vi "NurseStationMain.vi"() -> ()   [LabVIEW 2015]
uses:
  TypeDef/SelectedRoom.ctl
  LVClasses/Flags/ColorFlags.ctl
  TypeDef/RoomSelFromMap.ctl
  TypeDef/Flags_RoomNumber.ctl
  LVClasses/Room/Room.lvclass/Room.ctl
  TypeDef/State Cluster.ctl
  LVClasses/Room/Room.lvclass
  LVRestAPI/TypeDef/FGVAction.ctl
  LVClasses/Room/Read Flags.lvclass.vi
  LVClasses/Room/Read Room Number.vi
  LVClasses/Flags/Flags.lvclass
  LVRestAPI/RestApi.lvlib
panel:
  in  "Tab Control":enum32{"Main View", "Reports", "Debug"}(tab)
  out "Rooms":T1[](array[typedef])
  in  "New Request":bool
  out "Selected Room":T3={"Room Number"=0, "RoomNumFlags"={"Flag State"=[1, 3, 5, 7]}, "BedVacant"=FALSE, "InRoomPersonnel"=[], "RoomRequests"=[]}
  in  "SelRoom101":T4
  in  "SelRoom102":T4
  in  "SelRoom103":T4
  in  "stop":bool
  in  "ClearRequest":bool
  in  "ReqIndex":i32
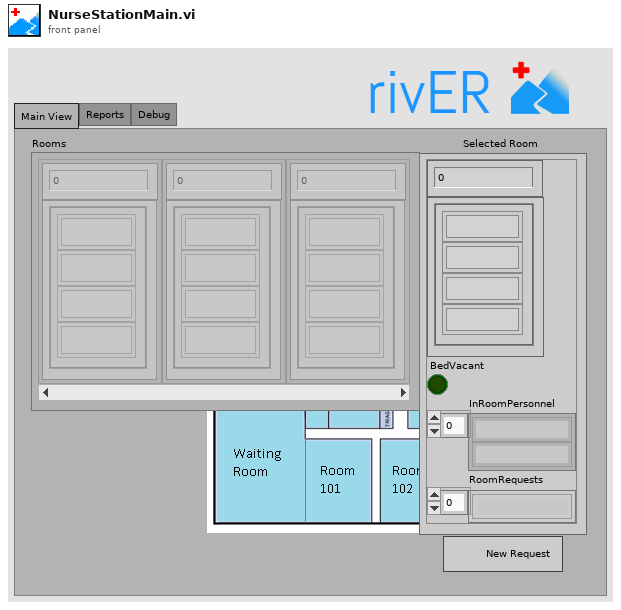
[diagram p1: front panel]
types:
  T1 = typedef "Flags_RoomNumber.ctl" = cluster{"Room Number":i32, "RoomNumFlags":T2}
  T2 = typedef "Flags.lvclass/ColorFlags.ctl" = cluster{"Flag State":u8[]}
  T3 = typedef "SelectedRoom.ctl" = cluster{"Room Number":u8, "RoomNumFlags":T2, "BedVacant":bool, "InRoomPersonnel":string[], "RoomRequests":string[]}
  T4 = typedef "RoomSelFromMap.ctl" = bool
  T5 = typedef "EventsReference.ctl" = cluster{"Init":refnum<user-event>, "Refresh UI":refnum<user-event>}
  T6 = typedef "FGVAction.ctl" = enum16{"Get", "Set"}
  T7 = typedef "State Cluster.ctl" = cluster{"Room Array":refnum<class "Room.lvclass">[], "Selected Room":u32}
  T8 = typedef "LVPoint32TypeDef.ctl" = cluster{"Horizontal":i32, "Vertical":i32}
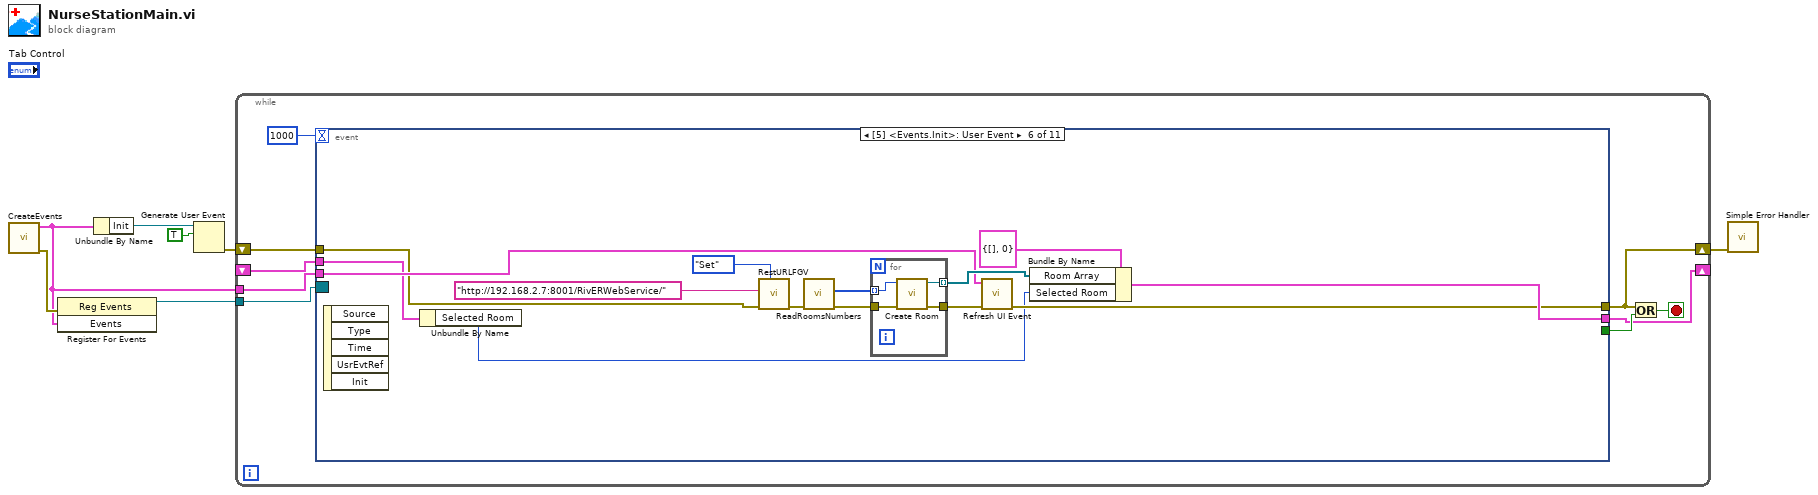
[diagram p0: block diagram]
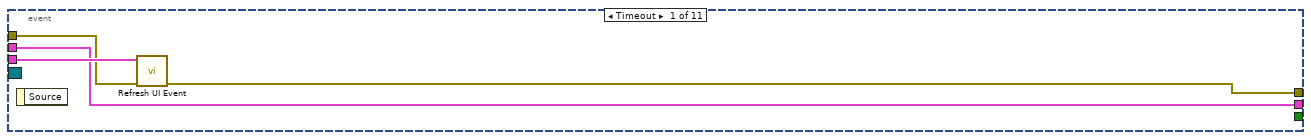
[diagram p2: hidden frame]
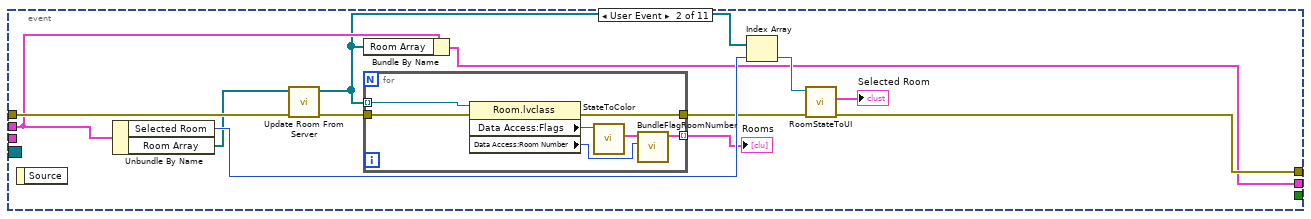
[diagram p3: hidden frame]
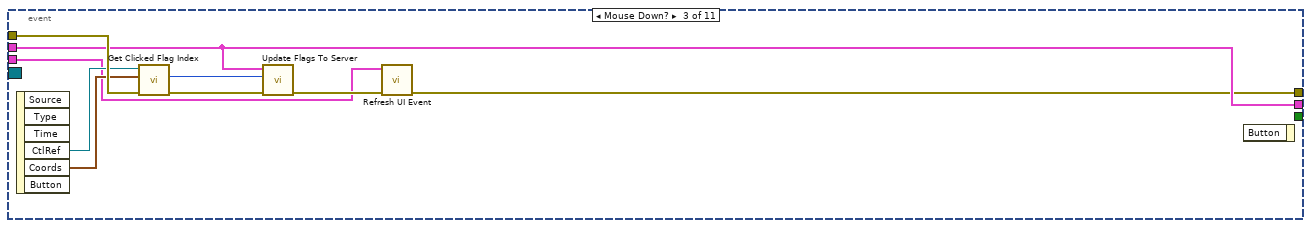
[diagram p4: hidden frame]
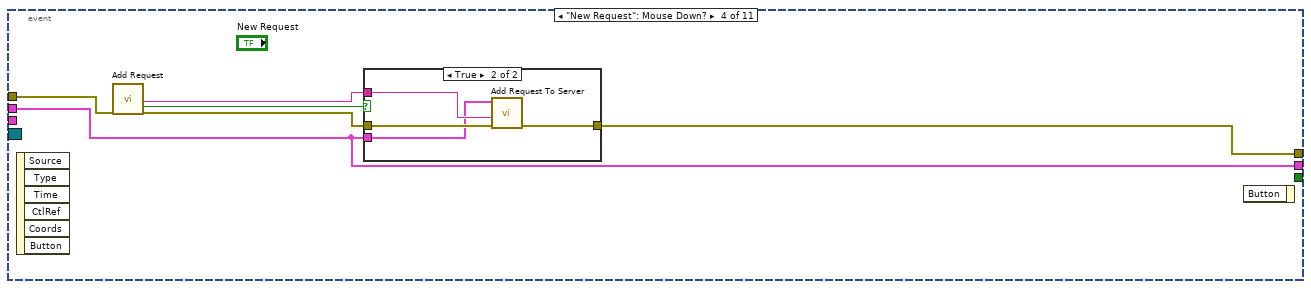
[diagram p5: hidden frame]
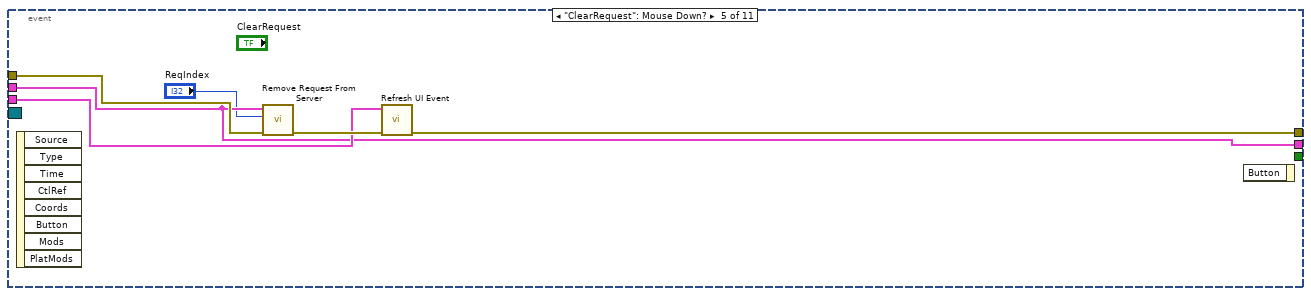
[diagram p7: hidden frame]
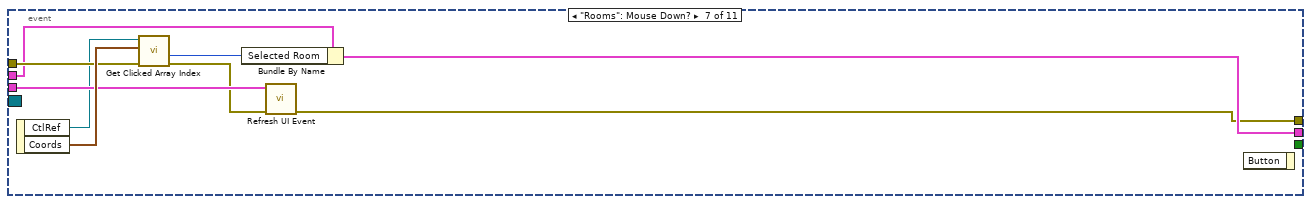
[diagram p8: hidden frame]
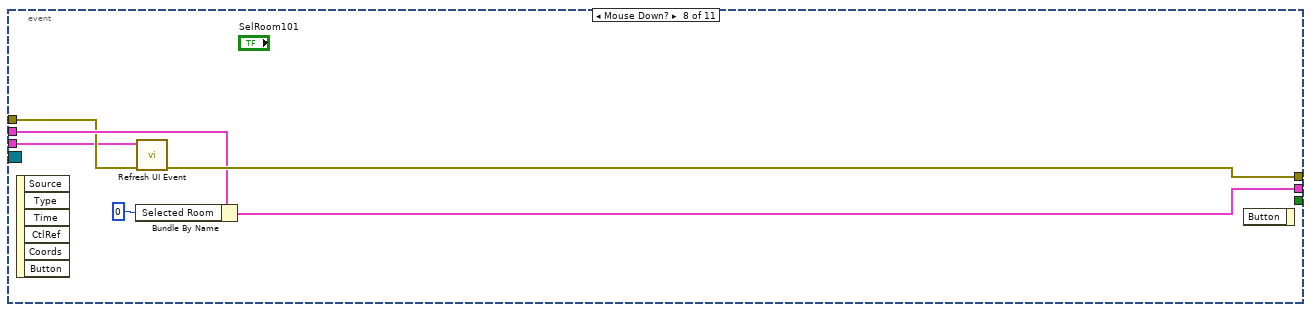
[diagram p9: hidden frame]
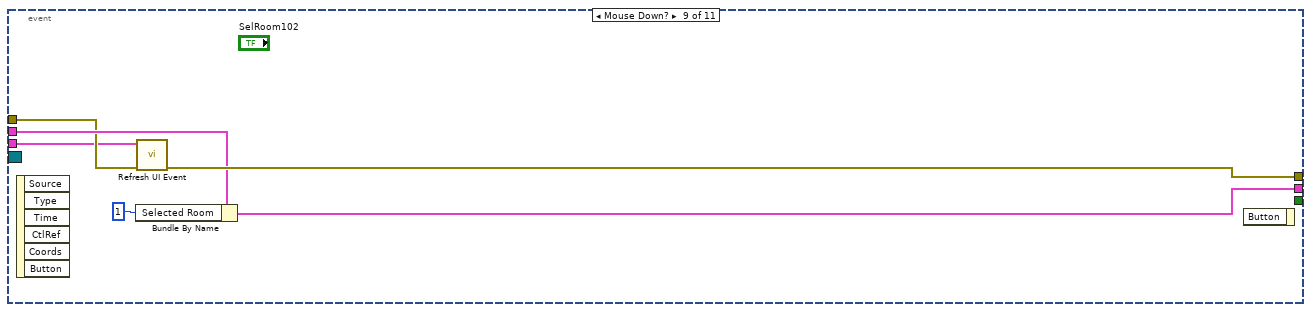
[diagram p10: hidden frame]
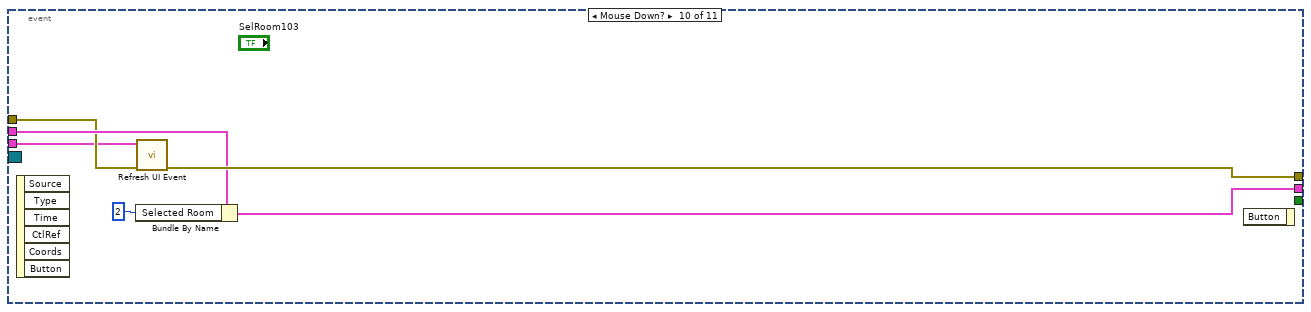
[diagram p11: hidden frame]
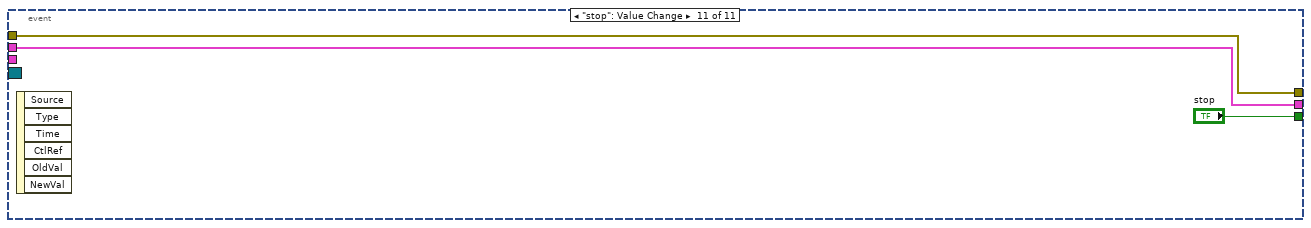
[diagram p12: hidden frame]
diagram:
  n1 = call "CreateEvents.vi"() -> ("error out"=w7:errorcluster, "Events"=w3:T5)  [unwired: 10 in]
  n2 = register-events(error in=w7, w3) -> (reference out=w6:refnum<event-registration>)  [unwired: 1 in, 1 out]
  n3 = Unbundle By Name(w3) -> ("Init"=w5:refnum<user-event>)
  n4 = Generate User Event(user event=w5, event data cluster=TRUE ("event data")) -> (error out=w2:errorcluster)  [unwired: 2 in, 1 out]
  n5 = while {
    shift-right: [w10] -> _
    shift-left: _ -> [w11]
    shift-right: [w13] -> w1
    shift-left: w2 -> [w16]
    tunnel: w6 -> [w12]
    tunnel: w3 -> [w9]
    stop <- w14 stop-if-true
    n6 = event shown="[5] <Events.Init>: User Event" {
      selector: w12 -> [_ _ _ _ _ _ _ _ _ _ _]
      dyn-events: _ -> [_ _ _ _ _ _ _ _ _ _ _]
      timeout: 1000 -> [_ _ _ _ _ _ _ _ _ _ _]
      tunnel: w16 -> [w19 w31 w48 w54 w65 w73 w91 w95 w101 w107 w112]
      tunnel: [w18 w29 w41 w49 w63 w74 w85 w98 w104 w110 w112] -> w13
      tunnel: [_ _ _ _ _ _ _ _ _ _ "stop"] -> w15
      tunnel: w11 -> [w17 w24 w43 w51 w61 w72 w90 w96 w102 w108 w111]
      tunnel: [w17 w22 w43 w51 w61 w78 w89 w97 w103 w109 w111] -> w10
      tunnel: w9 -> [w20 _ w40 _ w62 w76 w87 w94 w100 w106 _]
      event Timeout {
        n7 = event-data() -> ()  [unwired: 1 in, 1 out]
        n8 = call "Refresh UI Event.vi"("error in (no error)"=w19, "Events"=w20) -> ("error out"=w18:errorcluster)  [unwired: 9 in]
      }
      event User Event {
        n9 = event-data() -> ()  [unwired: 1 in, 1 out]
        n10 = Unbundle By Name(w24) -> ("Selected Room"=w32:u32, "Room Array"=w25:refnum<class "Room.lvclass">[])
        n11 = call "Update Room From Server.vi"("error in"=w31, "Room Array"=w25) -> ("error out"=w26:errorcluster, "Room Array Out"=w23:refnum<class "Room.lvclass">[])  [unwired: 8 in]
        n12 = Bundle By Name(cluster=w24, "Room Array"=w23) -> (w22:T7)
        n13 = for {
          tunnel: [w34] -> w21 mode=indexing
          tunnel: w23 -> [w38] mode=indexing
          tunnel: w26 -> [w37]
          tunnel: [w36] -> w30
          n14 = property class="Room.lvclass"(reference=w38, error in=w37) -> (error out=w36:errorcluster, "Data Access:Flags"=w39:refnum<class "Flags.lvclass">, "Data Access:Room Number"=w33:i32)  [unwired: 1 out]
          n15 = call "StateToColor.vi"("Flags in"=w39) -> ("RoomNumFlags"=w35:T2)  [unwired: 8 in, 2 out]
          n16 = call "BundleFlagRoomNumber.vi"("Room Number"=w33, "RoomNumFlags"=w35) -> ("Flags_RoomNum"=w34:T1)  [unwired: 9 in]
        }
        "Rooms" <- w21
        n17 = Index Array(array=w23, index=w32) -> (element=w27:refnum<class "Room.lvclass">)
        n18 = call "RoomStateToUI.vi"("error in"=w30, "Room In"=w27) -> ("error out"=w29:errorcluster, "Selected Room"=→"Selected Room":T3)  [unwired: 7 in, 1 out]
      }
      event Mouse Down? {
        n19 = event-data() -> ("CtlRef"=w46:refnum<vi>, "Coords"=w47:T8)  [unwired: 1 in, 4 out]
        n20 = call "Get Clicked Flag Index.vi"("error in"=w48, "Coordinates"=w47, "CtlRef"=w46) -> ("error out"=w45:errorcluster, "Row"=w42:i32)  [unwired: 6 in, 1 out]
        n21 = call "Update Flags To Server.vi"("error in"=w45, "Selected Flag"=w42, "State Cluster"=w43) -> ("error out"=w44:errorcluster)  [unwired: 8 in]
        n22 = call "Refresh UI Event.vi"("error in (no error)"=w44, "Events"=w40) -> ("error out"=w41:errorcluster)  [unwired: 9 in]
        n23 = event-data() -> ()  [unwired: 2 in, 1 out]
      }
      event "New Request": Mouse Down? {
        n24 = event-data() -> ()  [unwired: 1 in, 6 out]
        n25 = call "Add Request"("error in (no error)"=w54) -> ("Room Request"=w50:string, "OK"=w53:bool, "error out"=w52:errorcluster)  [unwired: 16 in]
        n26 = case shown="True" w53 {
          tunnel: w52 -> [w55 w59]
          tunnel: w51 -> [_ w56]
          tunnel: w50 -> [_ w57]
          tunnel: [w55 w58] -> w49
          frame False {
          }
          frame True {
            n27 = call "Add Request To Server.vi"("error in"=w59, "Room Request"=w57, "State Cluster"=w56) -> ("error out"=w58:errorcluster)  [unwired: 8 in]
          }
        }
        n28 = event-data() -> ()  [unwired: 2 in, 1 out]
      }
      event "ClearRequest": Mouse Down? {
        n29 = event-data() -> ()  [unwired: 1 in, 8 out]
        n30 = call "Remove Request From Server.vi"("error in"=w65, "ReqIndex"="ReqIndex", "State Cluster"=w61) -> ("error out"=w64:errorcluster)  [unwired: 8 in]
        n31 = call "Refresh UI Event.vi"("error in (no error)"=w64, "Events"=w62) -> ("error out"=w63:errorcluster)  [unwired: 9 in]
        n32 = event-data() -> ()  [unwired: 2 in, 1 out]
      }
      event User Event {
        n33 = event-data() -> ()  [unwired: 1 in, 5 out]
        n34 = Unbundle By Name(w72) -> ("Selected Room"=w71:u32)
        n35 = call "RestURLFGV.vi"("Action"=FGVAction."Set", "error in (no error)"=w73, "URL"="http://192.168.2.7:8001/RivERWebService/" ("url")) -> ("error out"=w67:errorcluster)  [unwired: 7 in, 1 out]
        n36 = call "ReadRoomsNumbers.vi"("error in (no error)"=w67) -> ("error out"=w66:errorcluster, "RoomNumbers"=w68:i32[])  [unwired: 9 in]
        n37 = for {
          tunnel: [w83] -> w75
          tunnel: [w82] -> w79 mode=indexing
          tunnel: w66 -> [w81]
          tunnel: w68 -> [w80] mode=indexing
          n38 = call "Create Room.vi"("error in"=w81, "Room Number"=w80) -> ("error out"=w83:errorcluster, "Room Ref"=w82:refnum<class "Room.lvclass">)  [unwired: 8 in]
        }
        n39 = call "Refresh UI Event.vi"("error in (no error)"=w75, "Events"=w76) -> ("error out"=w74:errorcluster)  [unwired: 9 in]
        n40 = Bundle By Name(cluster=T7 {"Room Array"=[], "Selected Room"=0} ("State Cluster"), "Room Array"=w79, "Selected Room"=w71) -> (w78:T7)
      }
      event "Rooms": Mouse Down? {
        n41 = event-data() -> ("CtlRef"=w84:refnum<vi>, "Coords"=w92:T8)  [unwired: 1 in]
        n42 = call "Get Clicked Array Index.vi"("error in"=w91, "Coordinates"=w92, "CtlRef"=w84) -> ("error out"=w86:errorcluster, "Column"=w88:i32)  [unwired: 6 in, 1 out]
        n43 = Bundle By Name(cluster=w90, "Selected Room"=w88) -> (w89:T7)
        n44 = call "Refresh UI Event.vi"("error in (no error)"=w86, "Events"=w87) -> ("error out"=w85:errorcluster)  [unwired: 9 in]
        n45 = event-data() -> ()  [unwired: 2 in, 1 out]
      }
      event Mouse Down? {
        n46 = event-data() -> ()  [unwired: 1 in, 6 out]
        n47 = Bundle By Name(cluster=w96, "Selected Room"=u32 0) -> (w97:T7)
        n48 = call "Refresh UI Event.vi"("error in (no error)"=w95, "Events"=w94) -> ("error out"=w98:errorcluster)  [unwired: 9 in]
        n49 = event-data() -> ()  [unwired: 2 in, 1 out]
      }
      event Mouse Down? {
        n50 = event-data() -> ()  [unwired: 1 in, 6 out]
        n51 = Bundle By Name(cluster=w102, "Selected Room"=u32 1) -> (w103:T7)
        n52 = call "Refresh UI Event.vi"("error in (no error)"=w101, "Events"=w100) -> ("error out"=w104:errorcluster)  [unwired: 9 in]
        n53 = event-data() -> ()  [unwired: 2 in, 1 out]
      }
      event Mouse Down? {
        n54 = event-data() -> ()  [unwired: 1 in, 6 out]
        n55 = Bundle By Name(cluster=w108, "Selected Room"=u32 2) -> (w109:T7)
        n56 = call "Refresh UI Event.vi"("error in (no error)"=w107, "Events"=w106) -> ("error out"=w110:errorcluster)  [unwired: 9 in]
        n57 = event-data() -> ()  [unwired: 2 in, 1 out]
      }
      event "stop": Value Change {
        n58 = event-data() -> ()  [unwired: 1 in, 6 out]
      }
    }
    n59 = Or(x=w13, y=w15) -> (x .or. y?=w14:bool)
  }
  n60 = call <vilib>:"Simple Error Handler.vi"("error in (no error)"=w1) -> ()  [unwired: 4 in, 5 out]
